vi "Read FE FF Frame.vi"(6 "Log Data?":bool, 8 "error in (no error)":errorcluster, 10 "CAN View Table":refnum<vi>, 11 "FE_FF_Decoder":T4={"Data Source"=enum."CSV File", "Frame Type"=enum."FE Frame", "Raw_Data?"=TRUE, "Config File Path"={"FE_FF_Data File"=path "D:/01_Vitesco/01_Projects/01-eDCU/10_LTT_Software/CAN Project/VAL SW Testing/Data/FE_FF_Data.csv", "FE_Frame_Details_File"=path "D:/01_Vitesco/01_Projects/01-eDCU/10_LTT_Software/CAN Project/VAL SW Testing/Data/FE_Frame_Details_eDCU.csv", "FF_Frame_Details_File"=path "D:/01_Vitesco/01_Projects/01-eDCU/10_LTT_Software/CAN Project/VAL SW Testing/Data/FF_Frame_Details_eDCU.csv"}, "CAN Init Data"={"XNET Interface"="", "Baud Rate"=0, "CAN:Termination"=0, "Echo Transmit?"=FALSE, "scope (normal)"=0}, "ResponseTimeout (S)"=0.0} {"CAN Init Data"."scope (normal)" items=["Normal", "Session Only", "Interface Only", "Session Only Blocking"]; "CAN Init Data"."CAN:Termination" items=["Off", "On"]; "CAN Init Data"."Baud Rate" format="%.0p"}) -> (0 "error out":errorcluster, 1 "RequestTimeout?":bool, 2 "PositiveResponse?":bool, 3 "Output Data":T5, 5 "Frame Detail":string[][](array[string]))   [LabVIEW 2023, in "GUI.lvlib" / "Diagnostic.lvlib" / "VAL_SW_Testing.lvlib"]
uses:
  VAL_SW_Testing.lvlib
  Ctrls/File Paths.ctl
  HardwareAbstractionLayer_LVOOP/CAN/CAN Lib/CAN_class/Ctrls/CAN Init Ctrl.ctl
  <vilib>/xnet/xnet.llb/XNET Control Scope.ctl
  HardwareAbstractionLayer_LVOOP/CAN/CAN Application Protocols/STP Protocol_class/Ctrls/STP Input Data.ctl
  HardwareAbstractionLayer_LVOOP/CAN/CAN Application Protocols/STP Protocol_class/Ctrls/STP CMD.ctl
  HardwareAbstractionLayer_LVOOP/Database/SQL Public VI/Control/DB Options.ctl
  <vilib>/Utility/file.llb/Read Delimited Spreadsheet (string).vi
  <userlib>/_OpenG.lib/array/array.llb/Filter 1D Array with Scalar (String)__ogtk.vi
  <userlib>/_OpenG.lib/array/array.llb/openg_array.lvlib
  HardwareAbstractionLayer_LVOOP/CAN/CAN Application Protocols/STP Protocol_class/STP Protocol.lvclass
  HardwareAbstractionLayer_LVOOP/Report/Report_class/Report.lvclass
  HardwareAbstractionLayer_LVOOP/Database/Database.lvclass
  HardwareAbstractionLayer_LVOOP/CAN/CAN Lib/CAN_class/CAN.lvclass
  HardwareAbstractionLayer_LVOOP/CAN/CAN Lib/Control/CAN Table.ctl
  HardwareAbstractionLayer_LVOOP/CAN/CAN Lib/CAN HAL Lib.lvlib
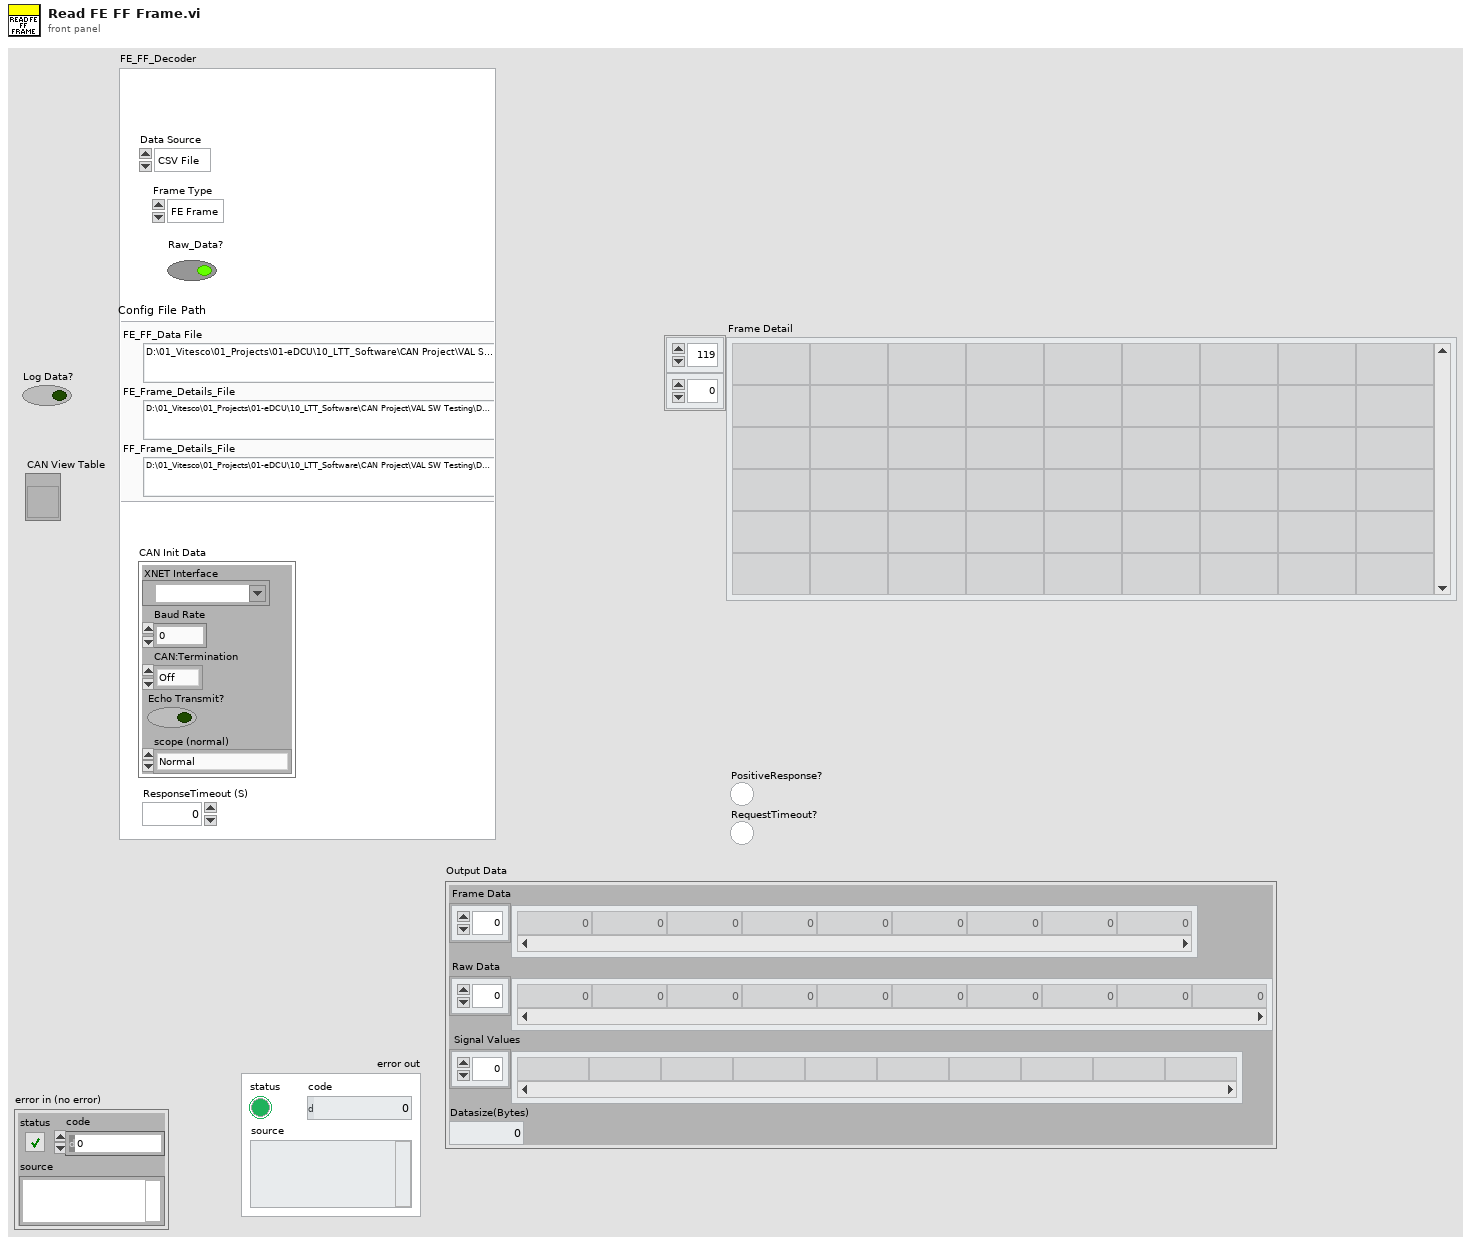
[diagram p1: front panel]
types:
  T1 = typedef "GUI.lvlib/Diagnostic.lvlib/VAL_SW_Testing.lvlib/File Paths.ctl" = cluster{"FE_FF_Data File":path, "FE_Frame_Details_File":path, "FF_Frame_Details_File":path}
  T2 = typedef "HardwareAbstractionLayer_LVOOP.lvlib/CAN HAL Lib.lvlib/CAN.lvclass/CAN Init Ctrl.ctl" = cluster{"XNET Interface":refnum<k21>, "Baud Rate":u64, "CAN:Termination":u32, "Echo Transmit?":bool, "scope (normal)":T3}
  T3 = typedef "XNET Control Scope.ctl" = u32
  T4 = cluster{"Data Source":enum16{"CSV File", "CAN"}, "Frame Type":enum16{"FE Frame", "FF Frame"}, "Raw_Data?":bool, "Config File Path":T1, "CAN Init Data":T2, "ResponseTimeout (S)":dbl}
  T5 = cluster{"Frame Data":u8[], "Raw Data":u64[], "Signal Values":string[], "Datasize(Bytes)":i32}
  T6 = typedef "HardwareAbstractionLayer_LVOOP.lvlib/Database.lvclass/DB Options.ctl" = enum16{"Init", "Select Data", "Insert Data", "Update Data", "Delete Data", "Execute Query", "Create Schema", "Create Table", "List Tables", "List Columns", "Close"}
  T7 = typedef "HardwareAbstractionLayer_LVOOP.lvlib/CAN Application Protocols Lib.lvlib/STP Protocol.lvclass/STP CMD.ctl" = u8
  T8 = typedef "HardwareAbstractionLayer_LVOOP.lvlib/CAN Application Protocols Lib.lvlib/STP Protocol.lvclass/STP Input Data.ctl" = cluster{"TxID":u32, "RxID":u32, "CMD":T7, "RQ Data":u8[], "+veResponseCode":u8, "ResponseTimeout (S)":dbl}
  T9 = typedef "HardwareAbstractionLayer_LVOOP.lvlib/CAN Application Protocols Lib.lvlib/STP Protocol.lvclass/STP Output Data.ctl" = cluster{"ResponseData":u8[], "ResponseData(ASCII)":string, "PositiveResponse?":bool, "STP Error":T10}
  T10 = typedef "HardwareAbstractionLayer_LVOOP.lvlib/CAN Application Protocols Lib.lvlib/STP Protocol.lvclass/STP Error Cluster.ctl" = cluster{"Status":bool, "Code":u8, "Error":string, "Description":string}
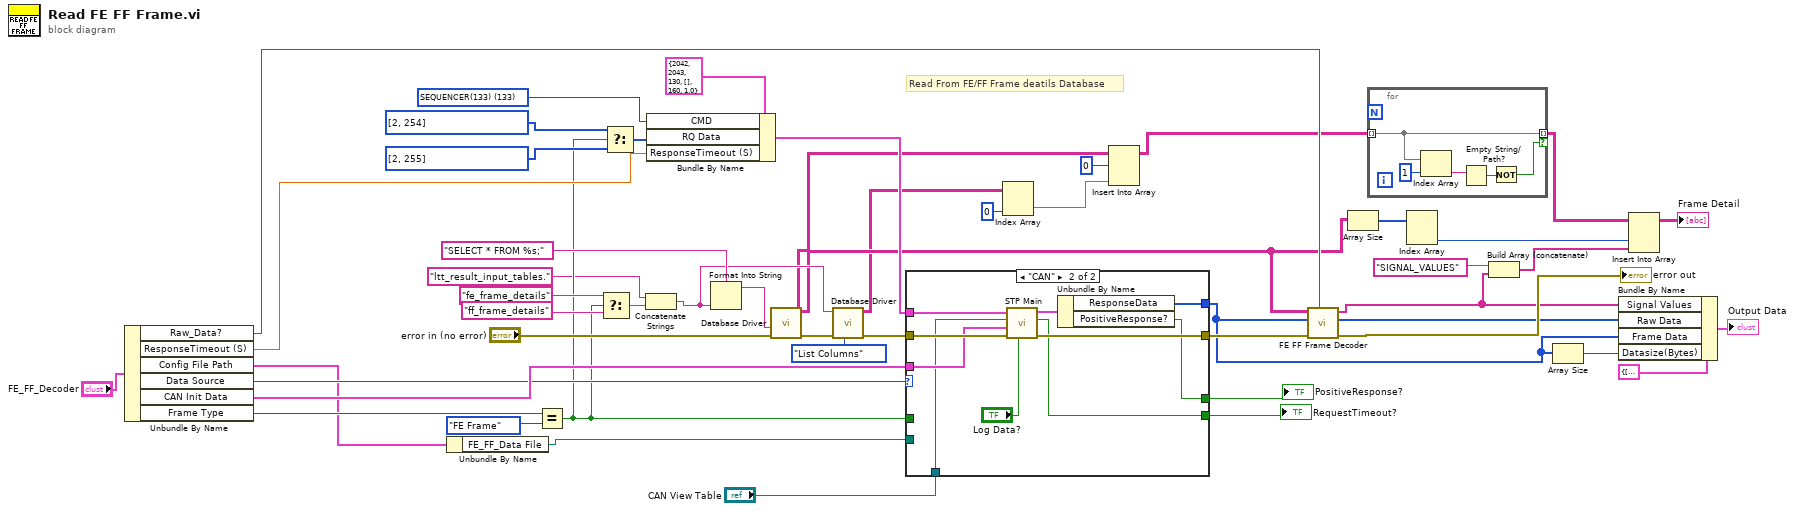
[diagram p0: block diagram]
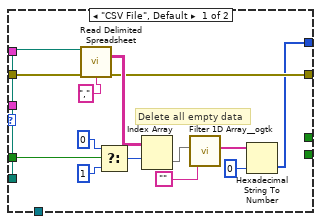
[diagram p2: hidden frame]
diagram:
  w46 = T7 133 items=["TSW_VERSION(130)"=130, "WAIT_EVENT(132)"=132, "SEQUENCER(133)"=133, "CONFIG_ECU(151)"=151, "TEST_CORE (152)"=152, "TEST_WATCHDOG (153)"=153, "TEST_MONITORING (154)"=154, "READ_MEMORY (162)"=162, "WRITE_ERASE_MEMORY (164)"=164, "COMM_EXTERNAL (190)"=190, "COMM_INTERNAL (195)"=195, "GET_ANALOG_INPUT (210)"=210, "GET_DIGITAL_INPUT (211)"=211, "GET_FREQUENCY_INPUT (212)"=212, "TEST_INPUT_STRUCTURE (214)"=214, "GENERATE_OUTPUT_SIGNAL (220)"=220, "GENERATE_SYNCHRONIZED_OUTPUT_SIGNALS (221)"=221, "eDCU_Specific (250)"=250] ("CMD")
  # "Read From FE/FF Frame deatils Database"
  n1 = Unbundle By Name("FE_FF_Decoder") -> ("Raw_Data?"=w19:bool, "ResponseTimeout (S)"=w29:dbl, "Config File Path"=w25:T1, "Data Source"=w27:enum16{"CSV File", "CAN"}, "CAN Init Data"=w28:T2, "Frame Type"=w26:enum16{"FE Frame", "FF Frame"})
  n2 = Unbundle By Name(w25) -> ("FE_FF_Data File"=w40:path)
  n3 = Equal?(x=w26, y=enum16{"FE Frame", "FF Frame"}."FE Frame" ("Frame Type")) -> (x = y?=w18:bool)
  n4 = Select(t="fe_frame_details", s=w18, f="ff_frame_details") -> (s? t:f=w15:string)
  n5 = Select(t=u8[] [2, 254] ("RQ Data"), s=w18, f=u8[] [2, 255] ("RQ Data")) -> (s? t:f=w50:u8[])
  n6 = Concatenate Strings("ltt_result_input_tables.", w15) -> (w13:string)
  n7 = Bundle By Name(cluster=T8 {"TxID"=2042, "RxID"=2043, "CMD"=130, "RQ Data"=[], "+veResponseCode"=160, "ResponseTimeout (S)"=1.0} ("STP Input Data"), "CMD"=w46, "RQ Data"=w50, "ResponseTimeout (S)"=w29) -> (w49:T8)
  n8 = Format Into String(format string="SELECT * FROM %s;" ("SQL query"), w13) -> (resulting string=w21:string)  [unwired: 2 in, 1 out]
  n9 = call "Database Driver.vi"("error in"="error in (no error)", "SQL query"=w21) -> ("error out"=w17:errorcluster, "data"=w7:string[][])  [unwired: 6 in, 2 out]
  n10 = call "Database Driver.vi"("Options"=DB_Options."List Columns", "error in"=w17, "table"=w13) -> ("error out"=w16:errorcluster, "data"=w6:string[][])  [unwired: 5 in, 2 out]
  n11 = case shown="\"CAN\"" w27 {
    tunnel: w40 -> [w64 _]
    tunnel: w16 -> [w63 w73]
    tunnel: w18 -> [w59 _]
    tunnel: [w57 w72] -> w34
    tunnel: w49 -> [_ w71]
    tunnel: [w53 w70] -> w32
    tunnel: w28 -> [_ w69]
    tunnel: [_ w68] -> w35
    tunnel: [_ w67] -> w36
    tunnel: "CAN View Table" -> [_ w65]
    frame "CSV File", Default {
      # "Delete all empty data"
      n12 = call-poly <vilib>:"Read Delimited Spreadsheet.vi"("file path (dialog if empty)"=w64, "error in (no error)"=w63, "delimiter (\\t)"="," ("delimiter (\\t)")) -> ("all rows"=w62:string[][], "error out"=w57:errorcluster)  [unwired: 7 in, 4 out]
      n13 = Select(t=0 ("index (row)"), s=w59, f=1 ("index (row)")) -> (s? t:f=w58:i32)
      n14 = Index Array(array=w62, index (row)=w58) -> (element=w56:string[])  [unwired: 1 in]
      n15 = call-poly <userlib>:"Filter 1D Array__ogtk.vi"("items to filter"="", "array"=w56) -> ("filtered array"=w52:string[])  [unwired: 4 in, 1 out]
      n16 = Hexadecimal String To Number(string=w52, default (0uL)=u8 0) -> (number=w53:u8[])  [unwired: 1 in, 1 out]
    }
    frame "CAN" {
      n17 = call "STP Main.vi"("Log Data?"="Log Data?", "error in (no error)"=w73, "CAN Init Data"=w69, "CAN View Table"=w65, "STP Input Data"=w71) -> ("error out"=w72:errorcluster, "RequestTimeout?"=w68:bool, "STP Output Data"=w74:T9)  [unwired: 4 in]
      n18 = Unbundle By Name(w74) -> ("ResponseData"=w70:u8[], "PositiveResponse?"=w67:bool)
    }
  }
  "PositiveResponse?" <- w36
  "RequestTimeout?" <- w35
  n19 = Index Array(array=w6, index (col)=0 ("disabled index (col)")) -> (element=w4:string[])  [unwired: 1 in]
  n20 = Insert Into Array(array=w7, index (row)=0, new element=w4) -> (w3:string[][])  [unwired: 1 in]
  n21 = call "FE FF Frame Decoder.vi"("Raw_Data?"=w19, "error in (no error)"=w34, "Frame Data"=w32, "Frame Detail"=w7) -> ("error out"=→"error out":errorcluster, "Raw Data"=w31:u64[], "Frame Detail With Value"=w11:string[])  [unwired: 5 in]
  n22 = Array Size(array=w7) -> (size(s)=w42:i32[])
  n23 = for {
    tunnel: w3 -> [w79] mode=indexing
    tunnel: [w79] -> w2 mode=indexing if=w76
    n24 = Index Array(array=w79, index=1) -> (element=w78:string)
    n25 = Empty String/Path?(string/path=w78) -> (empty?=w77:bool)
    n26 = Not(x=w77) -> (.not. x?=w76:bool)
  }
  n27 = Index Array(array=w42) -> (element #2=w41:i32)  [unwired: 2 in, 1 out]
  n28 = Build Array (concatenate)("SIGNAL_VALUES", w11) -> (w9:string[])
  n29 = Array Size(array=w32) -> (size(s)=w38:i32)
  n30 = Bundle By Name(cluster=T5 {"Frame Data"=[], "Raw Data"=[], "Signal Values"=[], "Datasize(Bytes)"=0} ("Output Data"), "Signal Values"=w11, "Raw Data"=w31, "Frame Data"=w32, "Datasize(Bytes)"=w38) -> (→"Output Data":T5)
  n31 = Insert Into Array(array=w2, index (col)=w41, new element=w9) -> (→"Frame Detail":string[][])  [unwired: 1 in]
